vi "Enable FDOT.vi"(7 "Enable FDOT (T: Enable)":bool=TRUE, 8 "error in (no error)":errorcluster, 11 "VISA resource name":refnum<visa-resource-name>) -> (0 "error out":errorcluster, 3 "VISA resource name out":refnum<visa-resource-name>)   [LabVIEW 2014, in "Agilent U2000 Series.lvlib"]
doc: "Enables or disables the use of the currently active sensor frequency-dependent offset table (CSET2). When a table has been selected and enabled, the sensor frequency-dependent offsets stored in it can be used by specifying the required frequency using the <b>Configure Correction Frequency.vi</b>."
uses:
  Agilent U2000 Series.lvlib
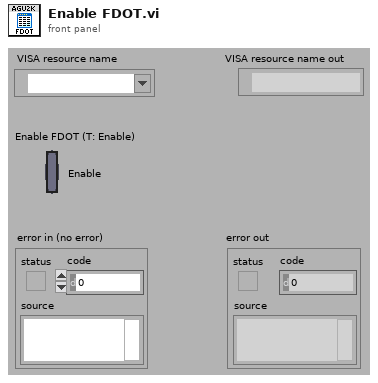
[diagram p1: front panel]
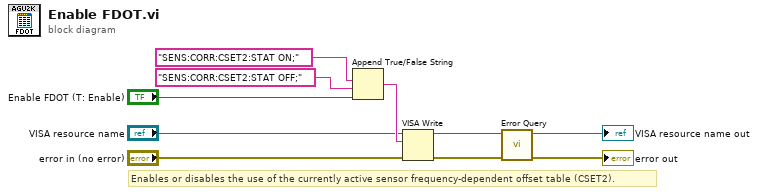
[diagram p0: block diagram]
diagram:
  # "Enables or disables the use of the currently active sensor frequency-dependent offset table (CSET2)."
  n1 = Append True/False String(1:"Enable FDOT (T: Enable)", 2:"SENS:CORR:CSET2:STAT OFF;", 3:"SENS:CORR:CSET2:STAT ON;") -> (0:w7:string)  [unwired: 1 out]
  n2 = VISA Write(VISA resource name="VISA resource name", write buffer=w7, error in (no error)="error in (no error)") -> (VISA resource name out=w4:refnum<visa-resource-name>, error out=w3:errorcluster)  [unwired: 1 out]
  n3 = call "Error Query.vi"("error in (no error)"=w3, "VISA resource name"=w4) -> ("error out"=→"error out":errorcluster, "VISA resource name out"=→"VISA resource name out":refnum<visa-resource-name>)  [unwired: 8 out]
